vi "Test_area-save.vi"() -> ()   [LabVIEW 2018]
panel:
  out "output cluster":T1
  out "Image":T2(plugin-control)
  in  "File Path out":path
  in  "Stop":bool
  in  "File Path in":path
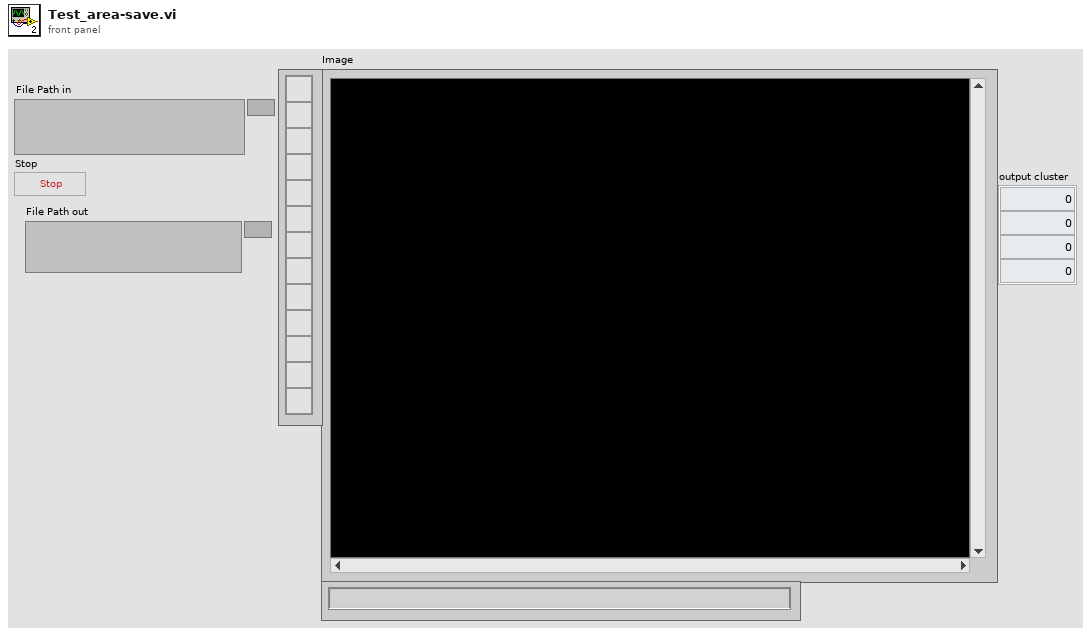
[diagram p1: front panel]
types:
  T1 = cluster{"Numeric":i32, "Numeric":i32, "Numeric":i32, "Numeric":i32}
  T2 = typedef "IMAQ Image.ctl" = refnum<image>
  T3 = cluster{"Global Rectangle":i32[], "Contours":cluster{"Contour Type":u32, "ROI Type":u32, "Points":i32[]}[]}
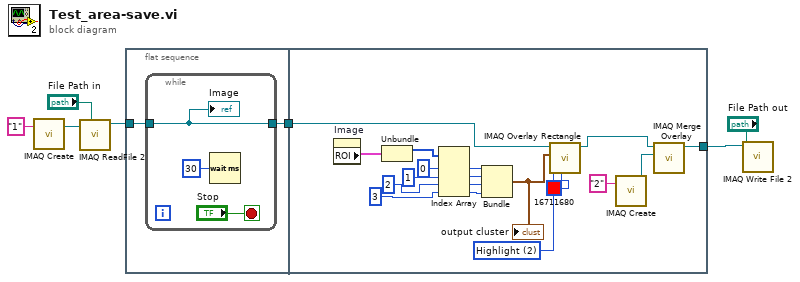
[diagram p0: block diagram]
diagram:
  n1 = call "IMAQ Create"("Image Name"="1") -> ("New Image"=w7:T2)  [unwired: 4 in, 1 out]
  n2 = call "IMAQ ReadFile 2"("File Path"="File Path in", "Image"=w7) -> ("Image Out"=w4:T2)  [unwired: 5 in, 4 out]
  n3 = flat-sequence {
    tunnel: w4 -> [w9]
    tunnel: [w8] -> w2
    tunnel: w2 -> [w19]
    tunnel: [w14] -> w1
    frame #0 {
      n4 = while {
        tunnel: w9 -> [w10]
        tunnel: [w10] -> w8
        stop <- "Stop" stop-if-true
        n5 = Wait (ms)(milliseconds to wait=u32 30) -> ()  [unwired: 1 out]
        "Image" <- w10
      }
    }
    frame #1 {
      w13 = u32 2 items=["Frame", "Fill", "Highlight"] ("Drawing Mode (Frame)")
      n6 = property on="Image" class="ImageControl"() -> ("ROI"=w22:T3)  [unwired: 2 in, 2 out]
      n7 = Unbundle(w22) -> ("Global Rectangle"=w27:i32[])  [unwired: 1 out]
      n8 = Index Array(array=w27, index #1=0 ("index"), index #2=1 ("index"), index #3=2 ("index"), index #4=3 ("index")) -> (element #1=w23:i32, element #2=w24:i32, element #3=w25:i32, element #4=w26:i32)
      n9 = Bundle(w23, w24, w25, w26) -> (w28:cluster{i32, i32, i32, i32})  [unwired: 1 in]
      "output cluster" <- w28
      n10 = call "IMAQ Overlay Rectangle"("Color"=u32 16711680, "Drawing Mode (Frame)"=w13, "Rectangle"=w28, "Image"=w19) -> ("Image Out"=w29:T2)  [unwired: 6 in, 1 out]
      n11 = call "IMAQ Create"("Image Name"="2") -> ("New Image"=w30:T2)  [unwired: 4 in, 1 out]
      n12 = call "IMAQ Merge Overlay"("Image Dst"=w30, "Image Src"=w29) -> ("Image Dst Out"=w14:T2)  [unwired: 8 in, 1 out]
    }
  }
  n13 = call-poly "IMAQ Write File 2"("File Path"="File Path out", "Image"=w1) -> ()  [unwired: 8 in, 2 out]
